vi "test_Count Monitor Data.vi"(6 "t_Monitor Enable":bool=TRUE, 8 "error in (no error)":errorcluster, 9 "t_ IO_St_Rd":u32, 10 "Monitor Data Cluster in":T1, 11 "Start or Stop Enable?":bool) -> (0 "error out":errorcluster, 2 "Monitor Data Cluster out":T1, 3 "Enable?":bool)   [LabVIEW 2016]
uses:
  FPGA/Typedefs/Monitor Data Cluster.ctl
  Host/Typedefs/IO Buffer Operation.ctl
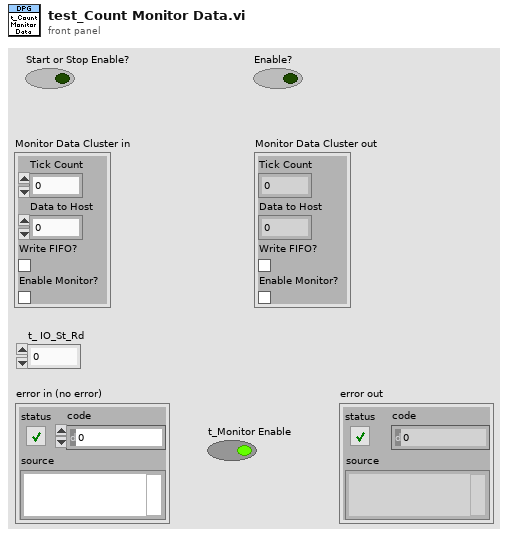
[diagram p1: front panel]
types:
  T1 = typedef "Monitor Data Cluster.ctl" = cluster{"Tick Count":u32, "Data to Host":u64, "Write FIFO?":bool, "Enable Monitor?":bool}
  T2 = typedef "IO Buffer Operation.ctl" = enum16{"Initialize", "Write IO Data_Rd", "Read IO Data_Rd", "Write IO Data_Wr", "Read IO Data_Wr", "Write  IO Data_Dir", "Read  IO Data_Dir", "Write Host to Target FIFO", "Read Host to Target FIFO", "Write Target to Host FIFO", "Read Target to Host FIFO", "Write Monitor Enable?", "Read Monitor Enable?", "Close"}
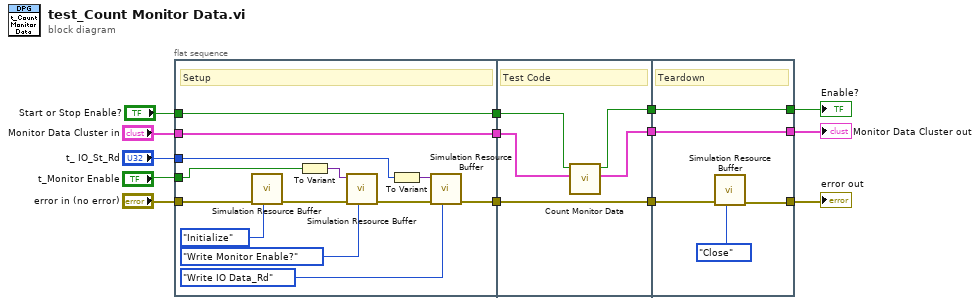
[diagram p0: block diagram]
diagram:
  n1 = flat-sequence {
    tunnel: "error in (no error)" -> [w17]
    tunnel: [w22] -> w12
    tunnel: "t_Monitor Enable" -> [w21]
    tunnel: "t_ IO_St_Rd" -> [w20]
    tunnel: "Start or Stop Enable?" -> [w19]
    tunnel: [w19] -> w9
    tunnel: "Monitor Data Cluster in" -> [w18]
    tunnel: [w18] -> w6
    tunnel: w12 -> [w32]
    tunnel: w9 -> [w31]
    tunnel: w6 -> [w30]
    tunnel: [w32] -> w5
    tunnel: [w29] -> w3
    tunnel: [w28] -> w2
    tunnel: [w36] -> w14
    tunnel: w5 -> [w37]
    tunnel: [w34] -> w4
    tunnel: w3 -> [w34]
    tunnel: [w33] -> w1
    tunnel: w2 -> [w33]
    frame #0 {
      # "Setup"
      n2 = call "Simulation Resource Buffer.vi"("IO Buffer Operation"=IO_Buffer_Operation."Initialize", "error in (no error)"=w17) -> ("error out"=w16:errorcluster)  [unwired: 7 in, 2 out]
      n3 = To Variant(anything=w21) -> (Variant=w25:variant)
      n4 = call "Simulation Resource Buffer.vi"("IO Buffer Operation"=IO_Buffer_Operation."Write Monitor Enable?", "error in (no error)"=w16, "Data in"=w25) -> ("error out"=w24:errorcluster)  [unwired: 6 in, 2 out]
      n5 = To Variant(anything=w20) -> (Variant=w23:variant)
      n6 = call "Simulation Resource Buffer.vi"("IO Buffer Operation"=IO_Buffer_Operation."Write IO Data_Rd", "error in (no error)"=w24, "Data in"=w23) -> ("error out"=w22:errorcluster)  [unwired: 6 in, 2 out]
    }
    frame #1 {
      # "Test Code"
      n7 = call "Count Monitor Data.vi"("Monitor Data Cluster in"=w30, "Start or Stop Enable?"=w31) -> ("Monitor Data Cluster out"=w28:T1, "Enable?"=w29:bool)  [unwired: 8 in]
    }
    frame #2 {
      # "Teardown"
      n8 = call "Simulation Resource Buffer.vi"("IO Buffer Operation"=IO_Buffer_Operation."Close", "error in (no error)"=w37) -> ("error out"=w36:errorcluster)  [unwired: 7 in, 2 out]
    }
  }
  "error out" <- w14
  "Enable?" <- w4
  "Monitor Data Cluster out" <- w1
